vi "Raster.vi"(4 "Draw Lines":bool, 6 "Line Colour":u32(colorbox)=4375295, 10 "Triangles Sorted":T1[](array[typedef]), 11 "Pixel Data in":u32[][](array[numeric])) -> (3 "Pixel Data out":u32[][](array[numeric]))   [LabVIEW 2020, in "3D.lvlib"]
uses:
  3D.lvlib
  Triangle 2D.ctl
  Point 2D.ctl
  Raster/Raster.lvlib
  Utility/Utility.lvlib
panel:
  out "Delta Time [s]":dbl format="%.3p"
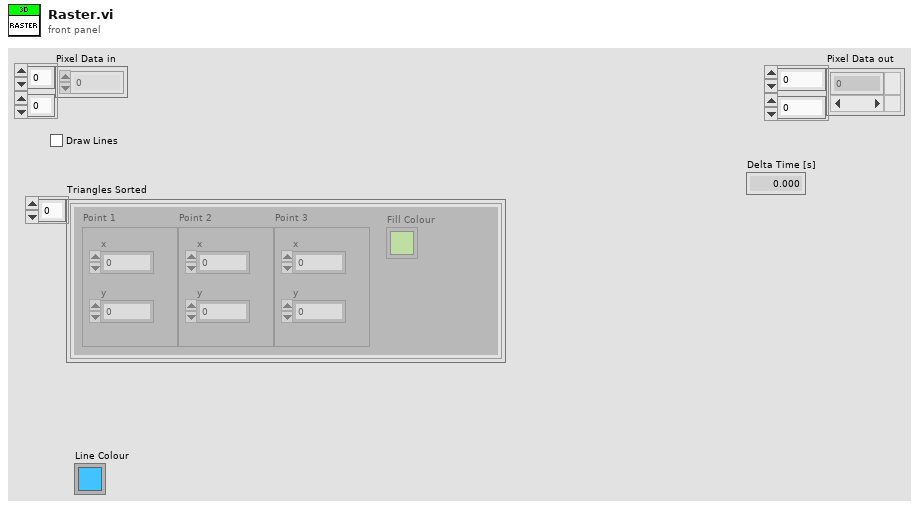
[diagram p1: front panel]
types:
  T1 = typedef "3D.lvlib/Triangle 2D.ctl" = cluster{"Point 1":T2, "Point 2":T2, "Point 3":T2, "Fill Colour":u32}
  T2 = typedef "3D.lvlib/Point 2D.ctl" = cluster{"x":sgl, "y":sgl}
  T3 = typedef "Raster.lvlib/Point 2D.ctl" = cluster{"x":i32, "y":i32}
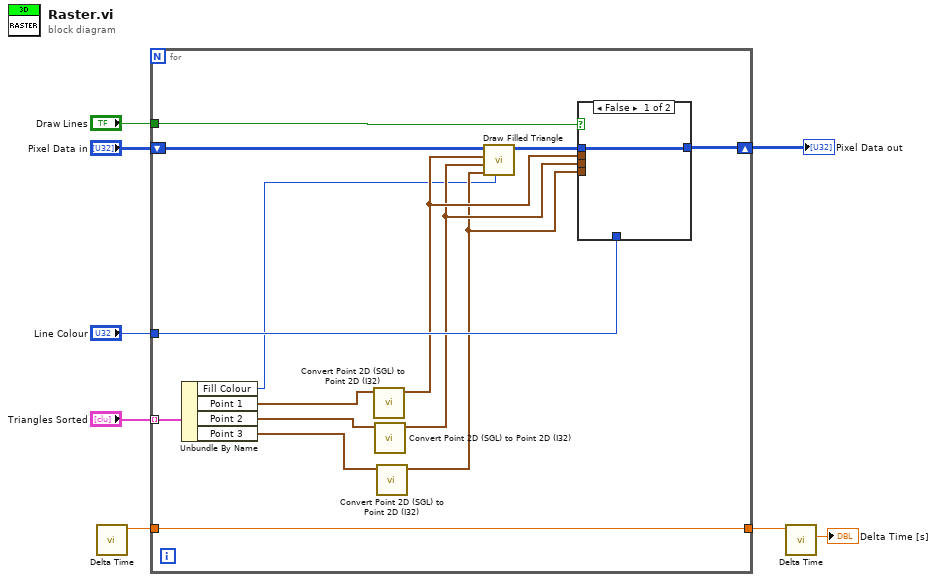
[diagram p0: block diagram]
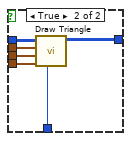
[diagram p2: hidden frame]
diagram:
  n1 = call "Delta Time.vi"() -> ("Relative Seconds Out"=w3:dbl)  [unwired: 10 in, 1 out]
  n2 = for {
    tunnel: "Line Colour" -> [w21]
    tunnel: "Triangles Sorted" -> [w18] mode=indexing
    shift-right: [w19] -> w6
    shift-left: "Pixel Data in" -> [w20]
    tunnel: "Draw Lines" -> [w10]
    tunnel: w3 -> [w9]
    tunnel: [w9] -> w2
    n3 = Unbundle By Name(w18) -> ("Fill Colour"=w11:u32, "Point 1"=w17:T2, "Point 2"=w16:T2, "Point 3"=w15:T2)
    n4 = call "Convert Point 2D (SGL) to Point 2D (I32).vi"("Point 2D (Float)"=w17) -> ("Point 2D (I32)"=w14:T3)  [unwired: 10 in]
    n5 = call "Convert Point 2D (SGL) to Point 2D (I32).vi"("Point 2D (Float)"=w16) -> ("Point 2D (I32)"=w13:T3)  [unwired: 10 in]
    n6 = call "Convert Point 2D (SGL) to Point 2D (I32).vi"("Point 2D (Float)"=w15) -> ("Point 2D (I32)"=w12:T3)  [unwired: 10 in]
    n7 = call "Draw Filled Triangle.vi"("Fill Colour"=w11, "Point 3"=w12, "Point 2"=w13, "Point 1"=w14, "Pixel Data in"=w20) -> ("Pixel Data out"=w22:u32[][])  [unwired: 6 in]
    n8 = case shown="False" w10 {
      tunnel: w22 -> [w23 w29]
      tunnel: w21 -> [_ w28]
      tunnel: [w23 w27] -> w19
      tunnel: w14 -> [_ w26]
      tunnel: w13 -> [_ w25]
      tunnel: w12 -> [_ w24]
      frame False {
      }
      frame True {
        n9 = call "Draw Triangle.vi"("Line Colour"=w28, "Point 3"=w24, "Point 2"=w25, "Point 1"=w26, "Pixel Data in"=w29) -> ("Pixel Data out"=w27:u32[][])  [unwired: 6 in]
      }
    }
  }
  "Pixel Data out" <- w6
  n10 = call "Delta Time.vi"("Relative Seconds In"=w2) -> ("Delta Time [s]"=→"Delta Time [s]":dbl)  [unwired: 9 in, 1 out]
